vi "Stop DMM - Current Mode.vi"(8 "error in (no error)":errorcluster, 11 "Async Data out":T1={"Hardware"={"Switch Device"="", "DMM Device"="", "DMM -> Switch Trigger"=0, "Switch -> DMM Trigger"=0, "Sample Interval (sec)"=0.0, "Current Samples"=0, "Current Limit"=1.2, "Current Resolution"=5.5, "Auto-Read"=FALSE, "Keep Values"=FALSE}, "Communication"={"Status Q"=refnum, "Command Q"=refnum, "Voltage FIFO"=refnum, "Voltage Buffer"=[], "Current FIFO"=refnum, "Current Buffer"=[], "Async Events"=refnum}} {"Hardware"."Current Resolution" items=["3 1/2"=3.5, "4 1/2"=4.5, "5 1/2"=5.5, "6 1/2"=6.5, "7 1/2"=7.5]; "Hardware"."Sample Interval (sec)" format="%.2f"}) -> (0 "error out":errorcluster)   [LabVIEW 2011, in "Switch-DMM Custom Device.lvlib"]
uses:
  Switch-DMM Custom Device.lvlib
  Controls/Async Data.ctl
  Controls/Hardware.ctl
  <instrlib>/niDMM/nidmm.llb/niDMM Resolution in Digits.ctl
  Controls/Communication.ctl
  Controls/Async Status.ctl
  Controls/Async State.ctl
  Controls/Async Command.ctl
  Controls/Async Events.ctl
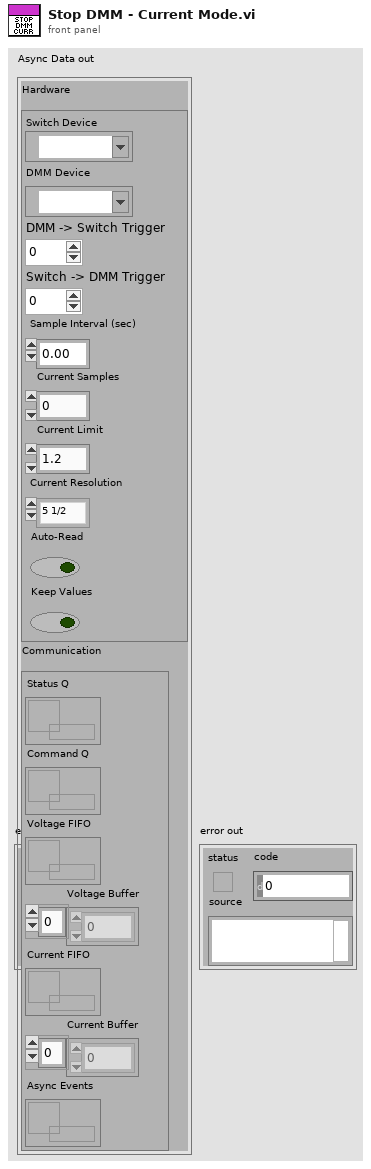
[diagram p1: front panel]
types:
  T1 = typedef "Switch-DMM Custom Device.lvlib/Async Data.ctl" = cluster{"Hardware":T2, "Communication":T4}
  T2 = typedef "Switch-DMM Custom Device.lvlib/Hardware.ctl" = cluster{"Switch Device":refnum<k15>, "DMM Device":refnum<k15>, "DMM -> Switch Trigger":u16, "Switch -> DMM Trigger":u16, "Sample Interval (sec)":dbl, "Current Samples":i32, "Current Limit":dbl, "Current Resolution":T3, "Auto-Read":bool, "Keep Values":bool}
  T3 = typedef "niDMM Resolution in Digits.ctl" = dbl
  T4 = typedef "Switch-DMM Custom Device.lvlib/Communication.ctl" = cluster{"Status Q":refnum<queue>, "Command Q":refnum<queue>, "Voltage FIFO":refnum<k33>, "Voltage Buffer":dbl[], "Current FIFO":refnum<k33>, "Current Buffer":dbl[], "Async Events":refnum<queue>}
  T5 = typedef "Switch-DMM Custom Device.lvlib/Async Command.ctl" = enum16{"None", "Start", "Set Cur Mode", "Req Volt Mode", "Set Volt Mode", "Read Volt", "Exit"}
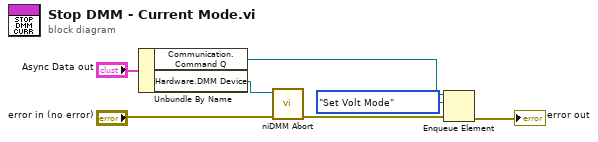
[diagram p0: block diagram]
diagram:
  n1 = Unbundle By Name("Async Data out") -> ("Communication.Command Q"=w2:refnum<queue>, "Hardware.DMM Device"=w4:refnum<k15>)
  n2 = call <instrlib>:"niDMM Abort.vi"("error in (no error)"="error in (no error)", "instrument handle"=w4) -> ("error out"=w5:errorcluster)  [unwired: 8 in, 1 out]
  n3 = Enqueue Element(queue=w2, element=Async_Command."Set Volt Mode", error in (no error)=w5) -> (error out=→"error out":errorcluster)  [unwired: 1 in, 2 out]
